vi "5.vi"() -> ()   [LabVIEW 2017]
panel:
  out "波形图":dbl[](graph)
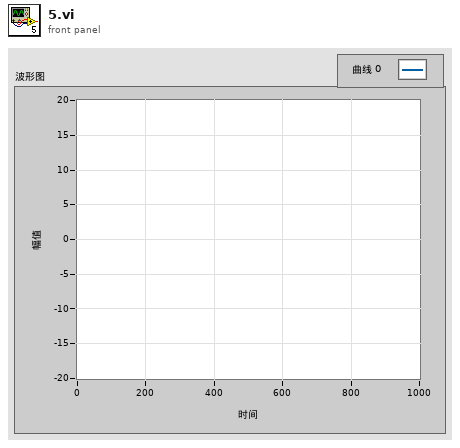
[diagram p1: front panel]
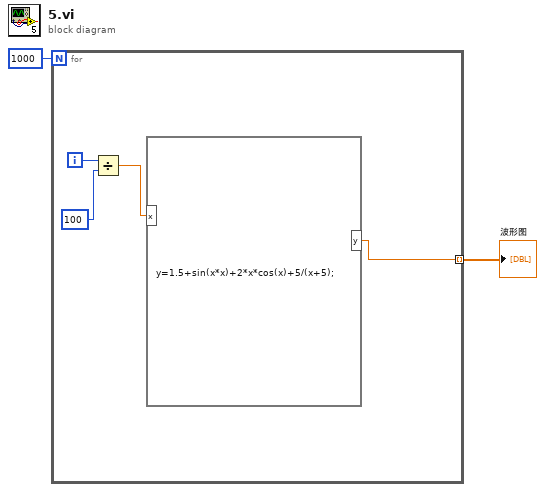
[diagram p0: block diagram]
diagram:
  n1 = for {
    N: 1000 -> [_]
    tunnel: [w3] -> w1 mode=indexing
    i -> [w6]
    n2 = Divide(x=w6, y=100) -> (x/y=w4:dbl)
    n3 = formula code="y=1.5+sin(x*x)+2*x*cos(x)+5/(x+5);"("x"=w4) -> ("y"=w3:dbl)
  }
  "波形图" <- w1
